vi "SHsUmrechnen-11-15.vi"(6 "TemperaturenSH[V]":dbl[](array[numeric]), 7 "SpannungenSH[V]":dbl[](array[numeric]), 9 "Traps/MachKoeff2":dbl[](array[numeric]), 10 "Traps/MachKoeff1":dbl[](array[numeric]), 11 "Traps/MachKoeff0":dbl[](array[numeric])) -> (2 "SpannungenSH[V]":fxp<+/-,16,4>[](array[numeric]) format="%.14g", 3 "TemperaturenSH[°C]":dbl[](array[numeric]))   [LabVIEW 2010]
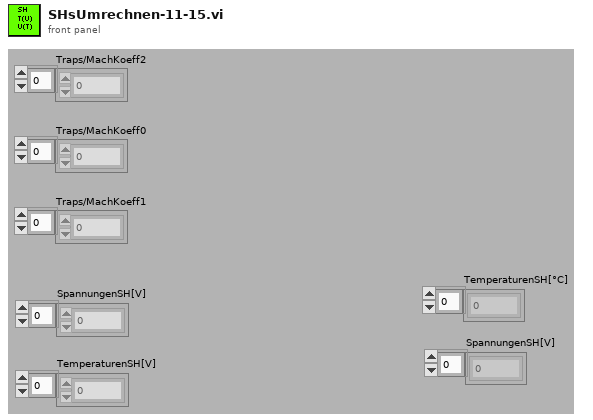
[diagram p1: front panel]
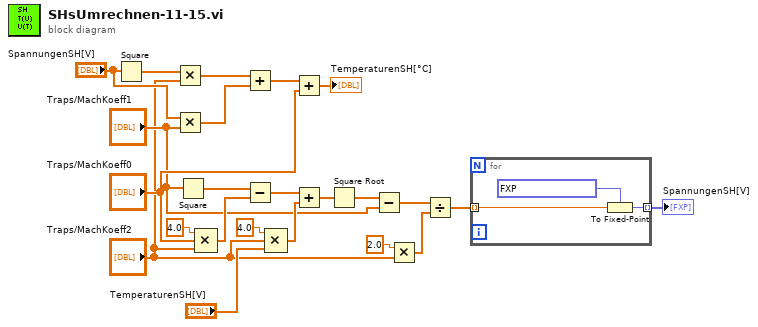
[diagram p0: block diagram]
diagram:
  n1 = Square(x="SpannungenSH[V]") -> (x^2=w20:dbl[])
  n2 = Multiply(x=w20, y="Traps/MachKoeff2") -> (x*y=w21:dbl[])
  n3 = Multiply(x="SpannungenSH[V]", y="Traps/MachKoeff1") -> (x*y=w22:dbl[])
  n4 = Square(x="Traps/MachKoeff1") -> (x^2=w13:dbl[])
  n5 = Compound Arithmetic op=MULTIPLY(4.0, "Traps/MachKoeff0", "Traps/MachKoeff2") -> (w12:dbl[])
  n6 = Add(x=w21, y=w22) -> (x+y=w23:dbl[])
  n7 = Subtract(x=w13, y=w12) -> (x-y=w11:dbl[])
  n8 = Compound Arithmetic op=MULTIPLY(4.0, "Traps/MachKoeff2", "TemperaturenSH[V]") -> (w10:dbl[])
  n9 = Add(x=w23, y="Traps/MachKoeff0") -> (x+y=→"TemperaturenSH[°C]":dbl[])
  n10 = Add(x=w11, y=w10) -> (x+y=w9:dbl[])
  n11 = Square Root(x=w9) -> (sqrt(x)=w8:dbl[])
  n12 = Subtract(x=w8, y="Traps/MachKoeff1") -> (x-y=w6:dbl[])
  n13 = Multiply(x=2.0, y="Traps/MachKoeff2") -> (x*y=w3:dbl[])
  n14 = Divide(x=w6, y=w3) -> (x/y=w2:dbl[])
  n15 = for {
    tunnel: w2 -> [w26] mode=indexing
    tunnel: [w25] -> w1 mode=indexing
    n16 = To Fixed-Point(fixed-point type=fxp<+/-,16,4> 0.0 ("USetp [V]Mach1"), number=w26) -> (fixed-point=w25:fxp<+/-,16,4>)
  }
  "SpannungenSH[V]" <- w1
